vi "SubVI_FilterDaqProcessorInfo.vi"(11 "Filtered Command Pairs":u8[][][](array[numeric])=[[[218, 0, 0, 0, 0, 0, 0, 0], [255, 8, 6, 0, 5, 0, 0, 80]]] format="%.0x") -> (1 "KeyByte_IdentificationField":u8 format="%.0b", 2 "Number of DAQ List Available":u8, 3 "CmdNotSupported":bool)   [LabVIEW 2019, in "XCP_DaqDtoId.lvlib" / "DAQList.lvclass"]
uses:
  DAQList.lvclass
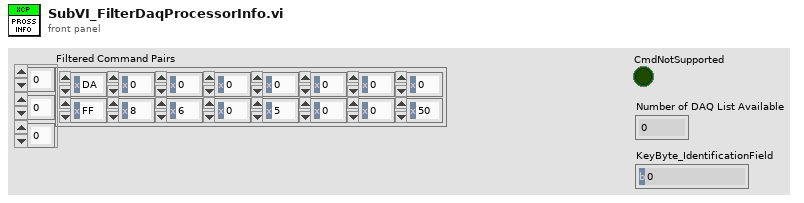
[diagram p1: front panel]
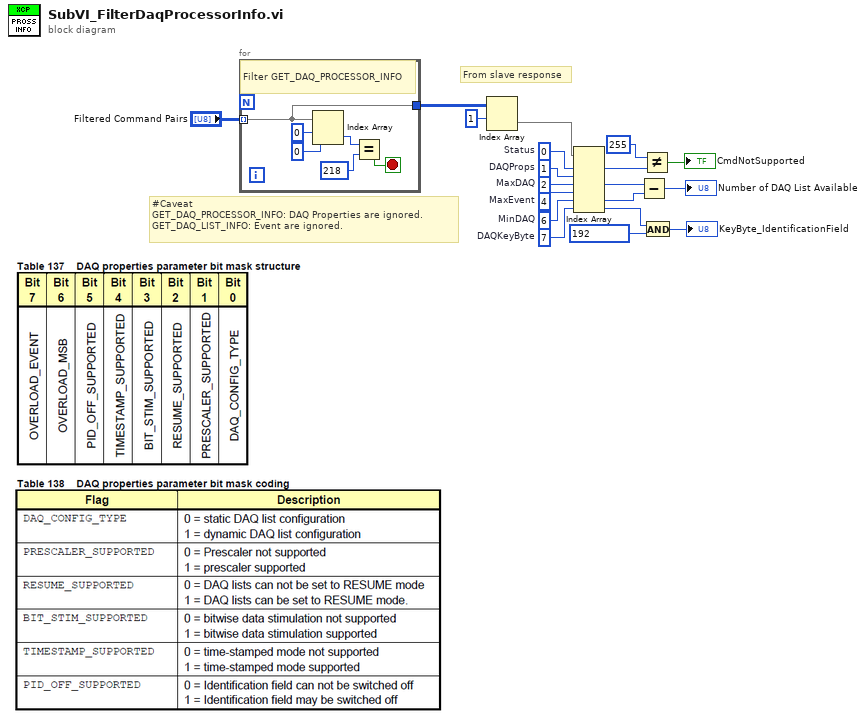
[diagram p0: block diagram]
diagram:
  w7 = 0  # Status
  w15 = 7  # DAQKeyByte
  w14 = 6  # MinDAQ
  w13 = 4  # MaxEvent
  w12 = 2  # MaxDAQ
  w11 = 1  # DAQProps
  # "#Caveat\nGET_DAQ_PROCESSOR_INFO: DAQ Properties are ignored.\nGET_DAQ_LIST_INFO: Event are ignored."
  # "From slave response"
  n1 = for {
    tunnel: "Filtered Command Pairs" -> [w21] mode=indexing
    tunnel: [w21] -> w8
    stop <- w20 stop-if-true
    # "Filter GET_DAQ_PROCESSOR_INFO"
    n2 = Index Array(array=w21, index (row)=0, index (col)=0 ("disabled index (col)")) -> (element=w23:u8)
    n3 = Equal?(x=w23, y=u8 218 ("element")) -> (x = y?=w20:bool)
  }
  n4 = Index Array(array=w8, index (row)=1) -> (element=w10:u8[])  [unwired: 1 in]
  n5 = Index Array(array=w10, index #1=w7, index #2=w11, index #3=w12, index #4=w13, index #5=w14, index #6=w15) -> (element #1=w6:u8, element #3=w16:u8, element #5=w17:u8, element #6=w3:u8)  [unwired: 2 out]
  n6 = Subtract(x=w16, y=w17) -> (x-y=→"Number of DAQ List Available":u8)
  n7 = Not Equal?(x=u8 255, y=w6) -> (x != y?=→"CmdNotSupported":bool)
  n8 = And(x=w3, y=u8 192) -> (x .and. y?=→"KeyByte_IdentificationField":u8)
